vi "Write Execution Time.vi"(8 "error in (no error)":errorcluster, 10 "Values in":dbl[](array[numeric]), 11 "Execution Unit in":refnum<class "Execution Unit.lvclass">) -> (0 "error out":errorcluster, 2 "Values out":dbl[](array[numeric]), 3 "Execution Unit out":refnum<class "Execution Unit.lvclass">)   [LabVIEW 2020, in "AIM ARINC 429 Engine.lvlib" / "Interfaces.lvlib" / "Execution Unit.lvclass"]
uses:
  Execution Unit.lvclass
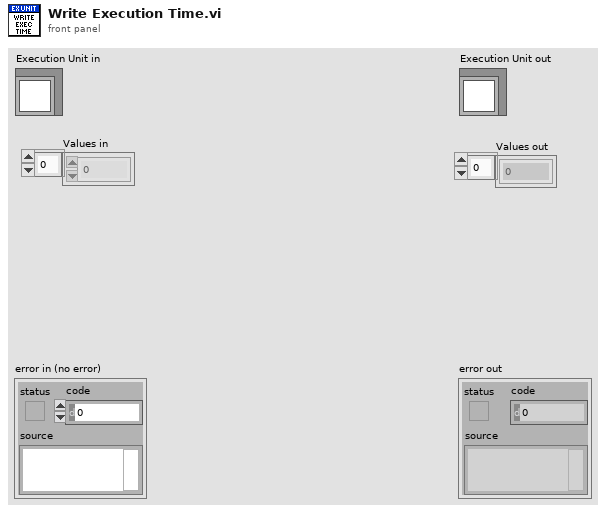
[diagram p1: front panel]
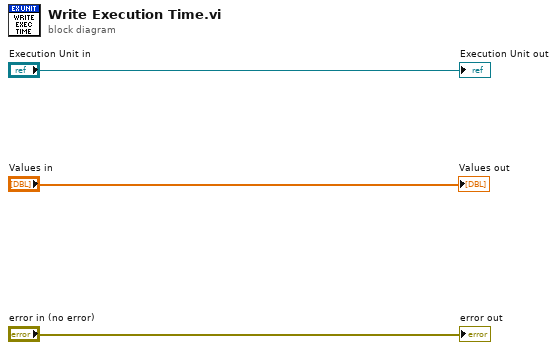
[diagram p0: block diagram]
diagram:
  "error out" <- "error in (no error)"
  "Execution Unit out" <- "Execution Unit in"
  "Values out" <- "Values in"
